vi "test broken method.vi"(8 "error in (no error)":errorcluster, 11 "TestCase in":refnum<class "VI Test Comparison.lvclass">) -> (0 "error out":errorcluster, 3 "TestCase out":refnum<class "VI Test Comparison.lvclass">)   [LabVIEW 2020, in "VI Test Comparison.lvclass"]
uses:
  VI Test Comparison.lvclass
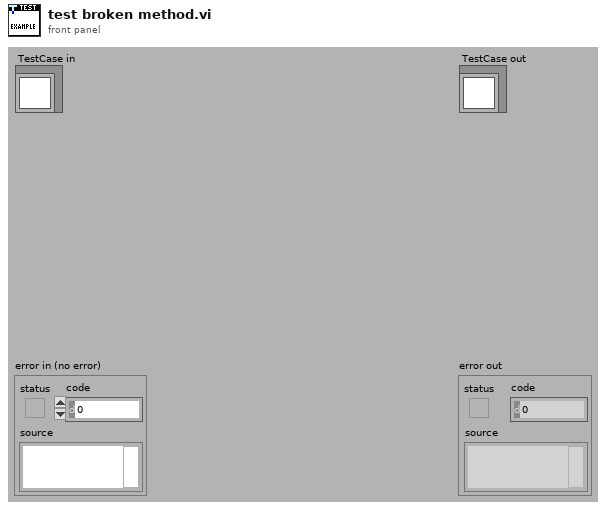
[diagram p1: front panel]
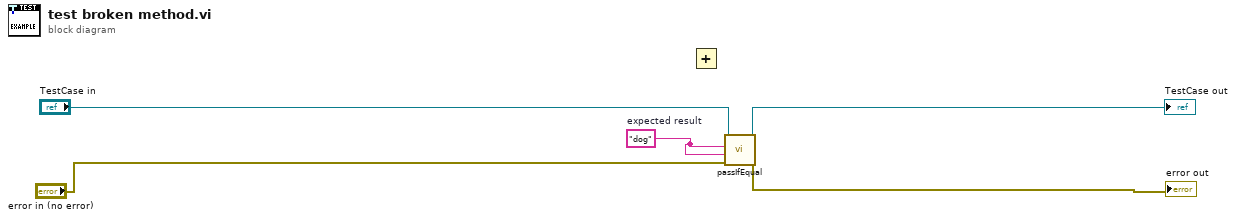
[diagram p0: block diagram]
diagram:
  w1 = "dog"  # expected result
  n1 = Add() -> ()  [unwired: 2 in, 1 out]
  n2 = call-dynamic "passIfEqual.vi"("error in (no error)"="error in (no error)", "y"=w1, "x"=w1, "TestCase in"="TestCase in") -> ("error out"=→"error out":errorcluster, "TestCase out"=→"TestCase out":refnum<class "VI Test Comparison.lvclass">)  [unwired: 6 in]
